vi "CRYMultitone Sub.vi"(4 "Max":dbl=1.0, 6 "Level Type":u16=1, 7 "Level In":dbl=1.0, 8 "dB ref":dbl=1.0, 9 "FAPS":T1(array[cluster]), 10 "samples":i32=1000, 11 "Fs":dbl=1000.0 format="%.2p") -> (3 "Multitone out":sgl[](array[numeric]) format="%.3f")   [LabVIEW 2013]
uses:
  <vilib>/Analysis/NI_AALBase.lvlib
  <vilib>/Analysis/NI_AALPro.lvlib
panel:
  in  "EQGain":dbl
  out "Waveform Graph 2":sgl[](graph)
  out "Waveform Graph":dbl[](graph)
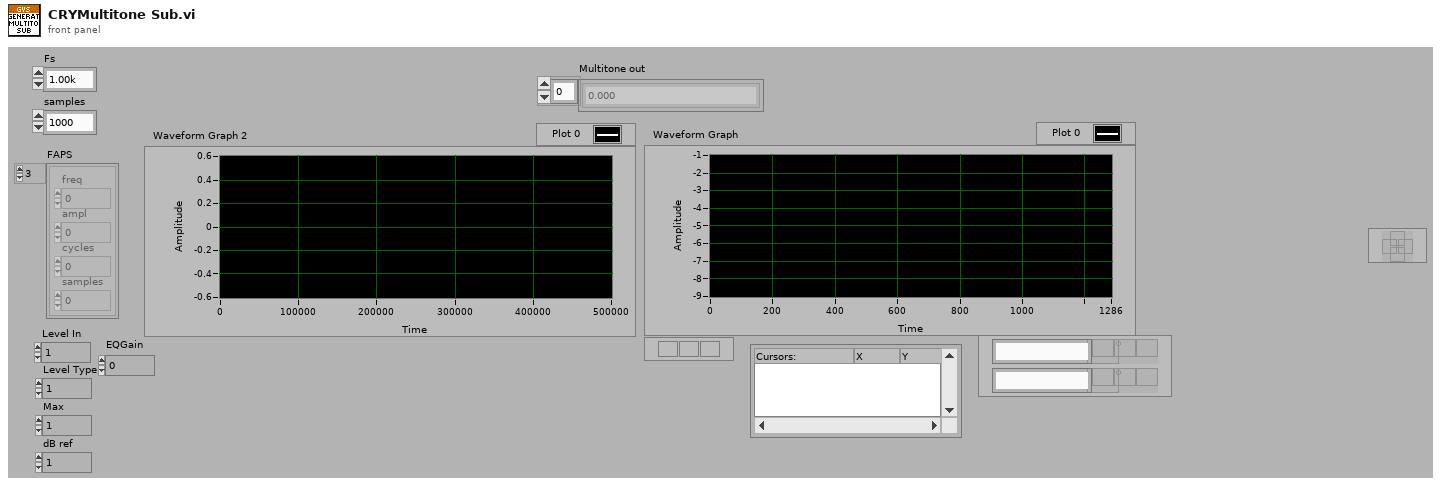
[diagram p1: front panel]
types:
  T1 = cluster{"freq":dbl, "ampl":dbl, "cycles":dbl, "samples":i32}[]
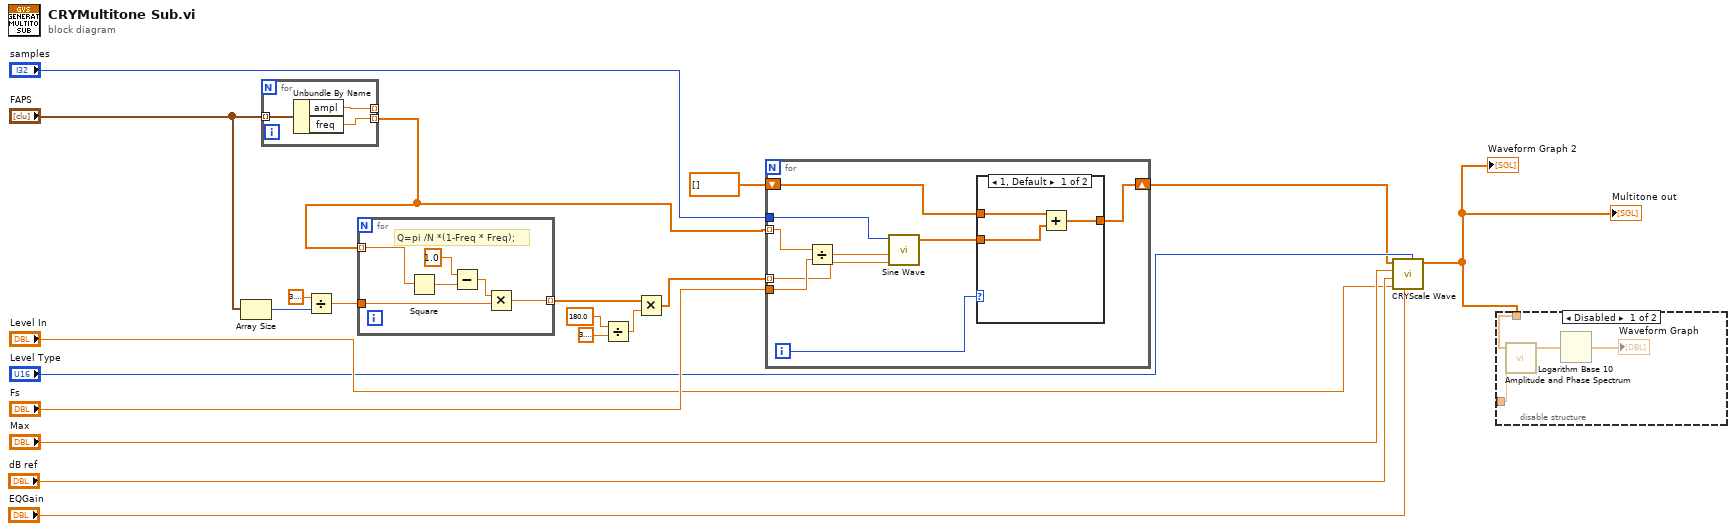
[diagram p0: block diagram]
diagram:
  n1 = Array Size(array="FAPS") -> (size(s)=w18:i32)
  n2 = for {
    tunnel: "FAPS" -> [w23] mode=indexing
    tunnel: [w22] -> w10 mode=indexing
    tunnel: [w21] -> _ mode=indexing
    n3 = Unbundle By Name(w23) -> ("ampl"=w21:dbl, "freq"=w22:dbl)
  }
  n4 = Divide(x=3.141592653589793, y=w18) -> (x/y=w17:dbl)
  n5 = for {
    tunnel: w10 -> [w27] mode=indexing
    tunnel: w17 -> [w25]
    tunnel: [w24] -> w14 mode=indexing
    # "Q=pi /N *(1-Freq * Freq);"
    n6 = Square(x=w27) -> (x^2=w28:dbl)
    n7 = Subtract(x=1.0 ("ampl"), y=w28) -> (x-y=w26:dbl)
    n8 = Multiply(x=w26, y=w25) -> (x*y=w24:dbl)
  }
  n9 = Divide(x=180.0, y=3.141592653589793) -> (x/y=w13:dbl)
  n10 = Multiply(x=w14, y=w13) -> (x*y=w12:dbl[])
  n11 = for {
    tunnel: w12 -> [w34] mode=indexing
    tunnel: "samples" -> [w38]
    tunnel: "Fs" -> [w36]
    tunnel: w10 -> [w35] mode=indexing
    shift-right: [w30] -> w2
    shift-left: dbl[] [] ("sine wave") -> [w31]
    i -> [w33]
    n12 = Divide(x=w35, y=w36) -> (x/y=w37:dbl)
    n13 = call <vilib>:"Sine Wave.vi"("samples"=w38, "frequency"=w37, "phase in"=w34) -> ("sine wave"=w32:dbl[])  [unwired: 2 in, 2 out]
    n14 = case shown="1, Default" w33 {
      tunnel: w32 -> [w40 w42]
      tunnel: w31 -> [w41 _]
      tunnel: [w39 w42] -> w30
      frame 1, Default {
        n15 = Add(x=w41, y=w40) -> (x+y=w39:dbl[])
      }
      frame 0 {
      }
    }
  }
  n16 = call "CRYScale Wave.vi"("Level Type"="Level Type", "EQGain"="EQGain", "Level"="Level In", "dB ref"="dB ref", "Max"="Max", "Wave"=w2) -> ("Scaled Wave"=w7:sgl[])  [unwired: 3 in, 2 out]
  "Multitone out" <- w7
  "Waveform Graph 2" <- w7
  n17 = disable-structure shown="Disabled" {
    disable-tunnel: _ -> [w46 _]
    disable-tunnel: w7 -> [w43 _]
    frame Disabled {
      n18 = call <vilib>:"Amplitude and Phase Spectrum.vi"("dt"=w46, "Signal (V)"=w43) -> ("Amp Spectrum Mag (Vrms)"=w45:dbl[])  [unwired: 1 in, 2 out]
      n19 = Logarithm Base 10(1:w45) -> (0:→"Waveform Graph":dbl[])
    }
    frame Enabled {
    }
  }
